vi "Multiply_HT.vi"(8 "Input Valid (T)":bool=TRUE, 9 "factor":u16, 10 "DDS sample":fxp<+/-,16,0>, 11 "Signal sample":fxp<+/-,16,16>) -> (0 "output valid":bool, 3 "Output":fxp<+/-,32,14>)   [LabVIEW 2018]
uses:
  <vilib>/rvi/FXPMathLib/FxpConvert/subVIs/nifxpmath_Convert_SimConfig.ctl
  <vilib>/fxp/LVFixedPointQuantizationPolicyTypeDef.ctl
  <vilib>/fxp/LVFixedPointOverflowPolicyTypeDef.ctl
  <vilib>/rvi/FXPMathLib/FxpConvert/simVIs/DllFxpConvertTemp_sub.vi
  <vilib>/rvi/FXPMathLib/FxpInterpret/XNode/nifxpmath_Interpret.xnode
  <vilib>/rvi/FXPMathLib/FxpConvert/XNode/nifxpmath_Convert.xnode
  <vilib>/rvi/FXPMathLib/FxpMul/XNode/nifxpmath_Multiplier.xnode
  <vilib>/rvi/FXPMathLib/sim/FxpSim.dll
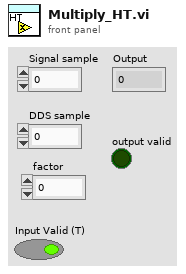
[diagram p1: front panel]
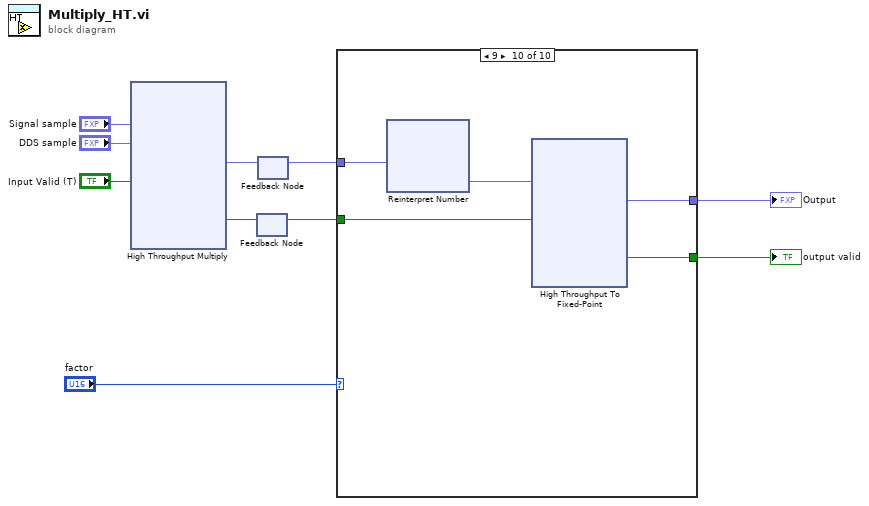
[diagram p0: block diagram]
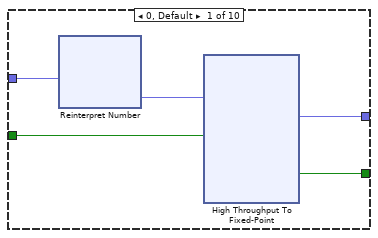
[diagram p2: hidden frame]
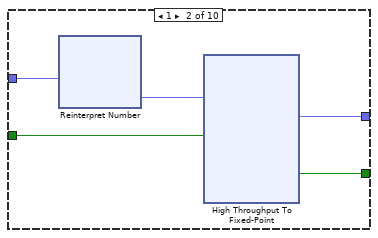
[diagram p3: hidden frame]
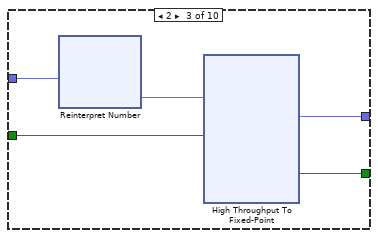
[diagram p4: hidden frame]
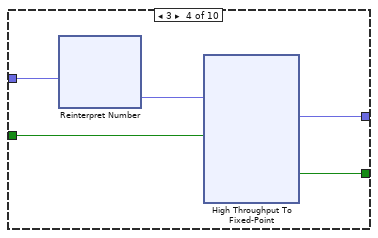
[diagram p5: hidden frame]
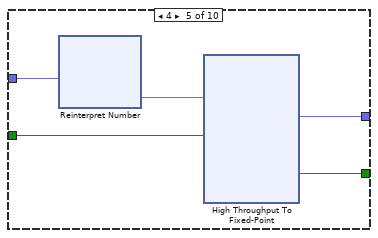
[diagram p6: hidden frame]
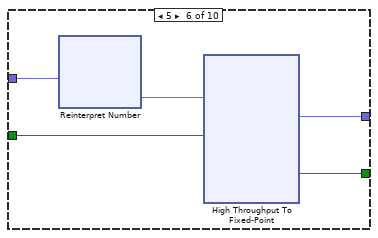
[diagram p7: hidden frame]
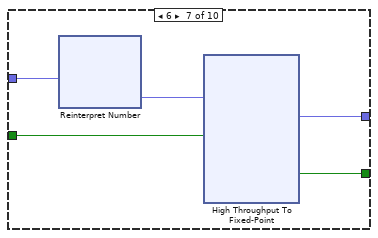
[diagram p8: hidden frame]
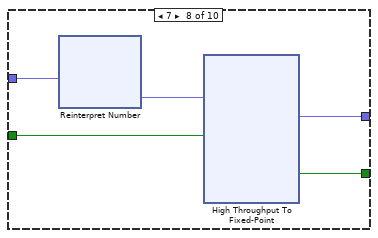
[diagram p9: hidden frame]
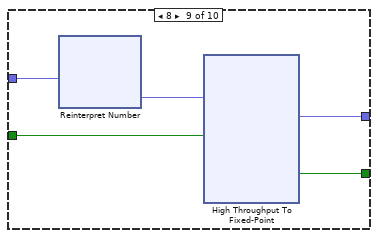
[diagram p10: hidden frame]
diagram:
  n1 = xnode ("High Throughput Multiply")("x"="Signal sample", "y"="DDS sample", "input valid"="Input Valid (T)") -> ("x*y"=w8:fxp<+/-,32,16>, "output valid"=w5:bool)  [unwired: 1 in, 1 out]
  n2 = feedback #1() -> (w4:bool)  [unwired: 1 in]
  n3 = feedback-in #1(w5) -> ()
  n4 = feedback #2() -> (w2:fxp<+/-,32,16>)  [unwired: 1 in]
  n5 = feedback-in #2(w8) -> ()
  n6 = case shown="9" "factor" {
    tunnel: [w15 w44 w73 w102 w131 w160 w189 w218 w247 w276] -> w6
    tunnel: w4 -> [w14 w43 w72 w101 w130 w159 w188 w217 w246 w275]
    tunnel: [w13 w42 w71 w100 w129 w158 w187 w216 w245 w274] -> w3
    tunnel: w2 -> [w12 w41 w70 w99 w128 w157 w186 w215 w244 w273]
    frame 0, Default {
      n7 = xnode "Reinterpret Number"("x"=w12) -> ("y"=w11:fxp<+/-,32,16>)
      n8 = xnode "High Throughput To Fixed-Point"("x"=w11, "input valid"=w14) -> ("y"=w15:fxp<+/-,32,14>, "output valid"=w13:bool)  [unwired: 1 in, 1 out]
    }
    frame 1 {
      n9 = xnode "Reinterpret Number"("x"=w41) -> ("y"=w40:fxp<+/-,32,17>)
      n10 = xnode "High Throughput To Fixed-Point"("x"=w40, "input valid"=w43) -> ("y"=w44:fxp<+/-,32,14>, "output valid"=w42:bool)  [unwired: 1 in, 1 out]
    }
    frame 2 {
      n11 = xnode "Reinterpret Number"("x"=w70) -> ("y"=w69:fxp<+/-,32,18>)
      n12 = xnode "High Throughput To Fixed-Point"("x"=w69, "input valid"=w72) -> ("y"=w73:fxp<+/-,32,14>, "output valid"=w71:bool)  [unwired: 1 in, 1 out]
    }
    frame 3 {
      n13 = xnode "Reinterpret Number"("x"=w99) -> ("y"=w98:fxp<+/-,32,19>)
      n14 = xnode "High Throughput To Fixed-Point"("x"=w98, "input valid"=w101) -> ("y"=w102:fxp<+/-,32,14>, "output valid"=w100:bool)  [unwired: 1 in, 1 out]
    }
    frame 4 {
      n15 = xnode "Reinterpret Number"("x"=w128) -> ("y"=w127:fxp<+/-,32,20>)
      n16 = xnode "High Throughput To Fixed-Point"("x"=w127, "input valid"=w130) -> ("y"=w131:fxp<+/-,32,14>, "output valid"=w129:bool)  [unwired: 1 in, 1 out]
    }
    frame 5 {
      n17 = xnode "Reinterpret Number"("x"=w157) -> ("y"=w156:fxp<+/-,32,21>)
      n18 = xnode "High Throughput To Fixed-Point"("x"=w156, "input valid"=w159) -> ("y"=w160:fxp<+/-,32,14>, "output valid"=w158:bool)  [unwired: 1 in, 1 out]
    }
    frame 6 {
      n19 = xnode "Reinterpret Number"("x"=w186) -> ("y"=w185:fxp<+/-,32,22>)
      n20 = xnode "High Throughput To Fixed-Point"("x"=w185, "input valid"=w188) -> ("y"=w189:fxp<+/-,32,14>, "output valid"=w187:bool)  [unwired: 1 in, 1 out]
    }
    frame 7 {
      n21 = xnode "Reinterpret Number"("x"=w215) -> ("y"=w214:fxp<+/-,32,23>)
      n22 = xnode "High Throughput To Fixed-Point"("x"=w214, "input valid"=w217) -> ("y"=w218:fxp<+/-,32,14>, "output valid"=w216:bool)  [unwired: 1 in, 1 out]
    }
    frame 8 {
      n23 = xnode "Reinterpret Number"("x"=w244) -> ("y"=w243:fxp<+/-,32,24>)
      n24 = xnode "High Throughput To Fixed-Point"("x"=w243, "input valid"=w246) -> ("y"=w247:fxp<+/-,32,14>, "output valid"=w245:bool)  [unwired: 1 in, 1 out]
    }
    frame 9 {
      n25 = xnode "Reinterpret Number"("x"=w273) -> ("y"=w272:fxp<+/-,32,25>)
      n26 = xnode "High Throughput To Fixed-Point"("x"=w272, "input valid"=w275) -> ("y"=w276:fxp<+/-,32,14>, "output valid"=w274:bool)  [unwired: 1 in, 1 out]
    }
  }
  "Output" <- w6
  "output valid" <- w3
